vi "Multiresolution Analysis - Image.vi"() -> ()   [LabVIEW 2023]
doc: "This example demonstrates how the Multiresolution Analysis 2D Express VI performs the discrete wavelet transform (DWT)-based multiresolution analysis. You can observe the image by using different resolutions. \n\nIn this example, the original image is a foil image. The peaks and valleys of the surface of the object in the original image are difficult to recognize visually. By using a low-high level of three in the Multiresolution Analysis Express VI, you can focus on the frequency bands in the column direction. You can observe the peaks and valleys of the surface more prominently in the coefficients at these frequency bands.\n\n<b>Instructions:</b>\n1) Run this VI.\n2) Compare the <b>Original Image</b> and the selected low-high frequency band at level three coefficients."
panel:
  out "Selected Coefficient":dbl[][](graph)
  out "Original Image":u8[][](graph)
  # "Overview: Demonstrates how the Multiresolution Analysis 2D Express VI performs the discrete wavelet transform (DWT)-based multiresolution analysis. You can observe the image by using different resolutions.\nRequirements: LabVIEW Full Development System, Advanced Signal Processing Toolkit\nInstructions: \n1. Run this VI.\n2. Compare the Original Image and the selected low-high frequency band at level three coefficients."
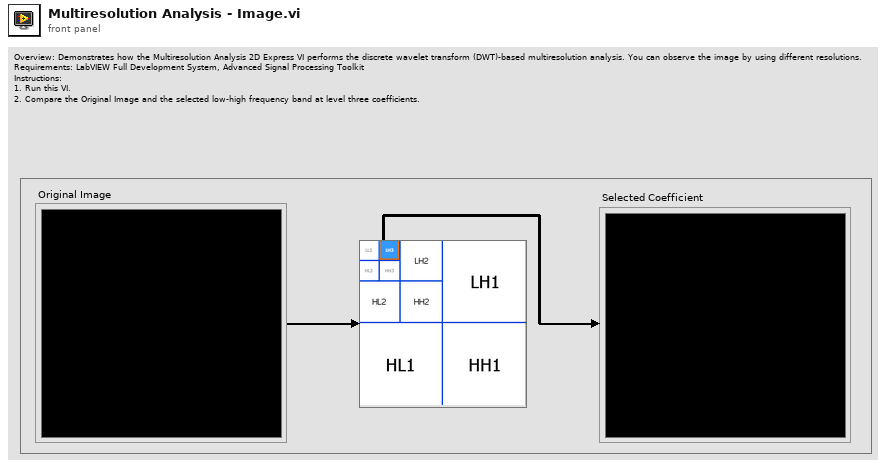
[diagram p1: front panel]
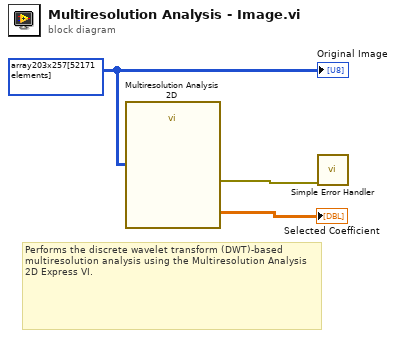
[diagram p0: block diagram]
diagram:
  w3 = u8[][] array203x257[52171 elements] ("Image")
  # "Performs the discrete wavelet transform (DWT)-based multiresolution analysis using the Multiresolution Analysis 2D Express VI."
  n1 = call "Multiresolution Analysis 2D"("Image"=w3) -> ("error out"=w1:errorcluster, "Selected Coefficients"=→"Selected Coefficient":dbl[][])  [unwired: 1 in, 8 out]
  n2 = call <vilib>:"Simple Error Handler.vi"("error in (no error)"=w1) -> ()  [unwired: 4 in, 5 out]
  "Original Image" <- w3
